vi "Attenuator Build Key Array for Config.vi"(8 "error in (no error)":errorcluster, 9 "DC Attenuation Test Parameters":T2={"Stimulus"={"ATT Stimulus"={"Normalize"=TRUE, "Value (dB)"=0.0}, "VNA Stimulus"={"Use Instrument Settings"=FALSE, "Blank Frequencies"=FALSE, "Sweep Type"=enum."Linear", "Sweep"={"Fstart"=500.0, "Fstop"=1500.0, "Units"=enum."MHz", "Points"=201}, "Power (dBm)"=999.0, "IFBW (Hz)"=-1.0, "Sweep Time (s)"=-1.0, "Calibration"={"State"=FALSE, "String"=""}}}, "Measurement"={"Step (dB)"=enum."0.25", "Start (dB)"=0.0, "Stop (dB)"=31.75}, "Limit"={"Maximum Error"=0.3}, "Normalization"={"Normalized?"=FALSE, "Normalization Values (dB)"=[]}} {"Stimulus"."VNA Stimulus"."Sweep Time (s)" format="%.3g"}, 10 "Key Array In":T11, 11 "Connection Refnum":T1) -> (0 "error out":errorcluster, 1 "$$INITCODE$$":string, 2 "Key Array Out":T11, 3 "Connection Refnum":T1)   [LabVIEW 2011]
uses:
  ITK EXT/utils/keyedarr.llb/Keyed Array.ctl
  TypeDefs/Attenuator Test Parameters.ctl
  TypeDefs/Attenuator Stimulus Parameters.ctl
  TypeDefs/Attenuator ATT Stimulus.ctl
  TypeDefs/Attenuator VNA Stimulus.ctl
  S Parameter/TypeDefs/SP Frequency Units.ctl
  TypeDefs/Attenuator VNA Calibration State.ctl
  TypeDefs/Attenuator Measurement Cluster.ctl
  TypeDefs/Attenuator Limit.ctl
  TypeDefs/Attenuator Calibration State.ctl
  Summitek EXT/ODBC/SQL Controls/Connection Refnum.ctl
  ITK EXT/utils/strutil.llb/Case Matching.ctl
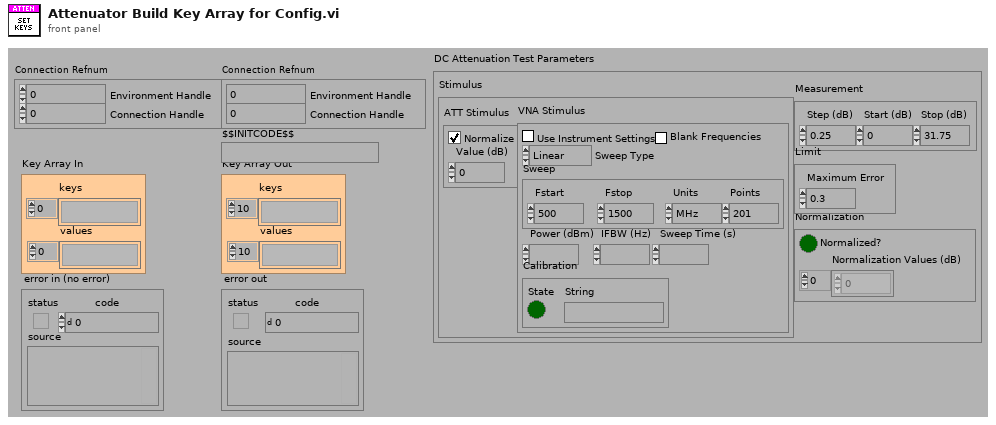
[diagram p1: front panel]
types:
  T1 = typedef "Connection Refnum.ctl" = cluster{"Environment Handle":i32, "Connection Handle":i32}
  T2 = typedef "Attenuator Test Parameters.ctl" = cluster{"Stimulus":T3, "Measurement":T8, "Limit":T9, "Normalization":T10}
  T3 = typedef "Attenuator Stimulus Parameters.ctl" = cluster{"ATT Stimulus":T4, "VNA Stimulus":T5}
  T4 = typedef "Attenuator ATT Stimulus.ctl" = cluster{"Normalize":bool, "Value (dB)":dbl}
  T5 = typedef "Attenuator VNA Stimulus.ctl" = cluster{"Use Instrument Settings":bool, "Blank Frequencies":bool, "Sweep Type":enum32{"Linear", "Logarithmic", "List", "Power", "CW"}, "Sweep":cluster{"Fstart":dbl, "Fstop":dbl, "Units":T6, "Points":i32}, "Power (dBm)":dbl, "IFBW (Hz)":dbl, "Sweep Time (s)":dbl, "Calibration":T7}
  T6 = typedef "SP Frequency Units.ctl" = enum16{"Hz", "kHz", "MHz", "GHz", "Points"}
  T7 = typedef "Attenuator VNA Calibration State.ctl" = cluster{"State":bool, "String":string}
  T8 = typedef "Attenuator Measurement Cluster.ctl" = cluster{"Step (dB)":enum16{"0.25", "0.50", "1.00"}, "Start (dB)":dbl, "Stop (dB)":dbl}
  T9 = typedef "Attenuator Limit.ctl" = cluster{"Maximum Error":dbl}
  T10 = typedef "Attenuator Calibration State.ctl" = cluster{"Normalized?":bool, "Normalization Values (dB)":dbl[]}
  T11 = typedef "Keyed Array.ctl" = cluster{"keys":string[], "values":string[]}
  T12 = typedef "Case Matching.ctl" = enum16{"a != A", "a == A", "system"}
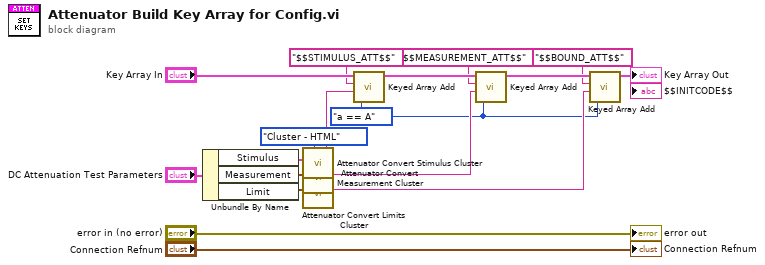
[diagram p0: block diagram]
diagram:
  w9 = enum16{"Cluster - HTML", "HTML - Cluster"}."Cluster - HTML" ("Conversion")
  w5 = Case_Matching."a == A" ("case matching (sensitive)")
  n1 = Unbundle By Name("DC Attenuation Test Parameters") -> ("Stimulus"=w10:T3, "Measurement"=w14:T8, "Limit"=w11:T9)
  n2 = call "Attenuator Convert Stimulus Cluster.vi"("Conversion"=w9, "Stimulus Cluster In"=w10) -> ("Stumulus HTML Out"=w3:string)  [unwired: 1 in, 5 out]
  n3 = call "Attenuator Convert Measurement Cluster.vi"("Conversion"=w9, "Measurements Cluster In"=w14) -> ("Measurements HTML Out"=w15:string)  [unwired: 1 in, 5 out]
  n4 = call "Attenuator Convert Limits Cluster.vi"("Conversion"=w9, "Limit Cluster In"=w11) -> ("Limits HTML Out"=w13:string)  [unwired: 2 in, 5 out]
  n5 = call "Keyed Array Add.vi"("case matching (sensitive)"=w5, "value"=w3, "key"="$$STIMULUS_ATT$$", "array in"="Key Array In") -> ("array out"=w6:T11)  [unwired: 3 out]
  n6 = call "Keyed Array Add.vi"("case matching (sensitive)"=w5, "value"=w15, "key"="$$MEASUREMENT_ATT$$", "array in"=w6) -> ("array out"=w17:T11)  [unwired: 3 out]
  n7 = call "Keyed Array Add.vi"("case matching (sensitive)"=w5, "value"=w13, "key"="$$BOUND_ATT$$", "array in"=w17) -> ("array out"=→"Key Array Out":T11)  [unwired: 3 out]
  "error out" <- "error in (no error)"
  "Connection Refnum" <- "Connection Refnum"
